vi "WriteL_thread.vi"(0 "val":u32, 1 "board_sel":u32, 2 "offset":u32) -> ()   [LabVIEW 2015]
uses:
  ESLSCDLL.dll
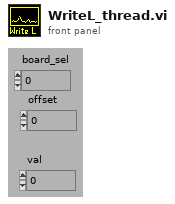
[diagram p1: front panel]
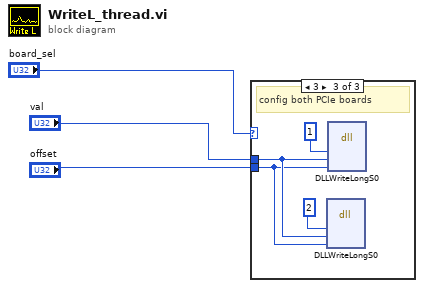
[diagram p0: block diagram]
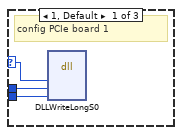
[diagram p2: hidden frame]
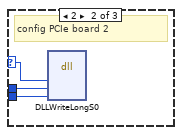
[diagram p3: hidden frame]
diagram:
  n1 = case shown="3" "board_sel" {
    selector: "board_sel" -> [w6 w9 _]
    tunnel: "val" -> [w5 w7 w11]
    tunnel: "offset" -> [w4 w8 w10]
    frame 1, Default {
      # "config PCIe board 1"
      n2 = dll-call lib="C:/ENTW/PCIE/lv64/board.vis/ESLSCDLL.dll" fn="DLLWriteLongS0"("drv"=w6, "DataByte"=w5, "PortOff"=w4) -> ()  [unwired: 7 in, 2 out]
    }
    frame 2 {
      # "config PCIe board 2"
      n3 = dll-call lib="C:/ENTW/PCIE/lv64/board.vis/ESLSCDLL.dll" fn="DLLWriteLongS0"("drv"=w9, "DataByte"=w7, "PortOff"=w8) -> ()  [unwired: 7 in, 2 out]
    }
    frame 3 {
      # "config both PCIe boards"
      n4 = dll-call lib="C:/ENTW/PCIE/lv64/board.vis/ESLSCDLL.dll" fn="DLLWriteLongS0"("drv"=u32 2, "DataByte"=w11, "PortOff"=w10) -> ()  [unwired: 7 in, 2 out]
      n5 = dll-call lib="C:/ENTW/PCIE/lv64/board.vis/ESLSCDLL.dll" fn="DLLWriteLongS0"("drv"=u32 1, "DataByte"=w11, "PortOff"=w10) -> ()  [unwired: 7 in, 2 out]
    }
  }
